vi "RespaceForSP.vi"(9 "Keep spaces?":bool, 11 "Code":string) -> (3 "Cleaned for SPIKE":string)   [LabVIEW 2020]
panel:
  out "spreadsheet string":string
  out "Array":i32[](array[numeric])
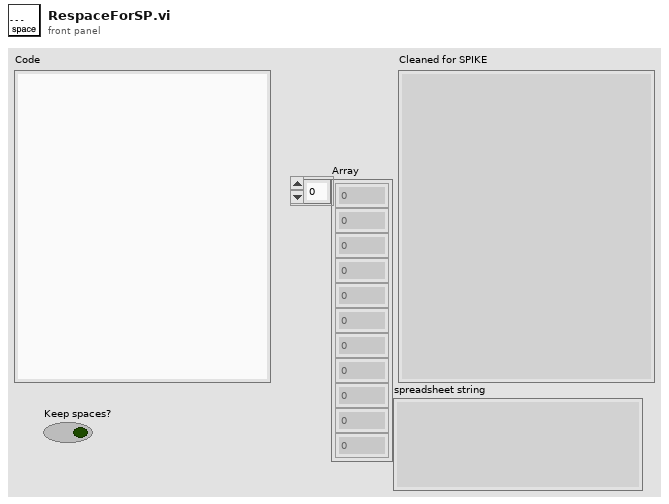
[diagram p1: front panel]
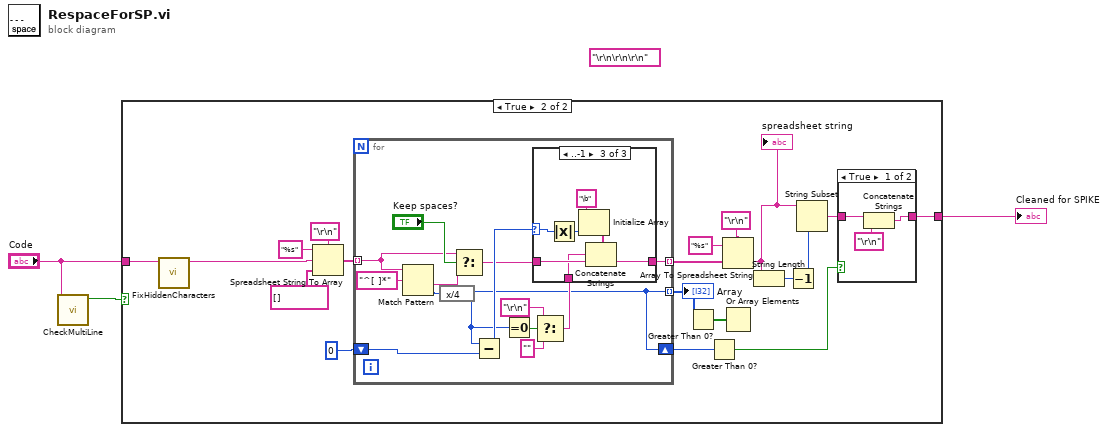
[diagram p0: block diagram]
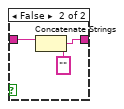
[diagram p3: hidden frame]
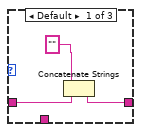
[diagram p4: hidden frame]
diagram:
  (unwired) "\r\n\r\n\r\n" ("replace string (\"\")")
  n1 = call "CheckMultiLine.vi"("Code"="Code") -> ("MultiLine?"=w1:bool)  [unwired: 10 in]
  n2 = case shown="True" w1 {
    tunnel: "Code" -> [w4 w23]
    tunnel: [w4 w14] -> w3
    frame False {
    }
    frame True {
      n3 = call "FixHiddenCharacters.vi"("String in"=w23) -> ("String out"=w5:string)  [unwired: 10 in]
      n4 = Spreadsheet String To Array(delimiter (Tab)="\r\n" ("replace string (\"\")"), format string="%s", spreadsheet string=w5, array type (2D Dbl)=string[] []) -> (array=w19:string[])
      n5 = for {
        tunnel: [w31] -> _ mode=indexing
        tunnel: w19 -> [w31] mode=indexing
        tunnel: [w34] -> w13 mode=indexing
        tunnel: [w40] -> w18 mode=indexing
        shift-right: [w34] -> w7
        shift-left: 0 ("offset past match") -> [w42]
        n6 = Match Pattern(string=w31, regular expression="^[ ]*") -> (after substring=w32:string, offset past match=w35:i32)  [unwired: 1 in, 2 out]
        n7 = expression code="x/4"(w35) -> (w34:i32)
        n8 = Select(t=w31, s="Keep spaces?", f=w32) -> (s? t:f=w30:string)
        n9 = Subtract(x=w34, y=w42) -> (x-y=w41:i32)
        n10 = Equal To 0?(x=w34) -> (x = 0?=w39:bool)
        n11 = Select(t="\r\n" ("replace string (\"\")"), s=w39, f="" ("replace string (\"\")")) -> (s? t:f=w36:string)
        n12 = case shown="..-1" w41 {
          selector: w41 -> [_ _ w52]
          tunnel: [w45 w47 w54] -> w40
          tunnel: w30 -> [w46 w47 w53]
          tunnel: w36 -> [_ _ w48]
          frame Default {
            n13 = Concatenate Strings("" ("replace string (\"\")"), w46) -> (w45:string)
          }
          frame 0 {
          }
          frame ..-1 {
            n14 = Absolute Value(x=w52) -> (abs(x)=w50:i32)
            n15 = Initialize Array("\b" ("replace string (\"\")"), w50) -> (w49:string[])
            n16 = Concatenate Strings(w49, w48, w53) -> (w54:string)
          }
        }
      }
      "Array" <- w13
      n17 = Greater Than 0?(x=w13) -> (x > 0?=w12:bool[])
      n18 = Greater Than 0?(x=w7) -> (x > 0?=w6:bool)
      n19 = Array To Spreadsheet String(delimiter (Tab)="\r\n" ("replace string (\"\")"), array=w18, 3:"%s" ("format string")) -> (spreadsheet string=w10:string)
      "spreadsheet string" <- w10
      n20 = Or Array Elements(Boolean array=w12) -> ()  [unwired: 1 out]
      n21 = String Length(string=w10) -> (length=w11:i32)
      n22 = Decrement(x=w11) -> (x-1=w8:i32)
      n23 = String Subset(string=w10, length (rest)=w8) -> (substring=w9:string)  [unwired: 1 in]
      n24 = case shown="True" w6 {
        tunnel: w9 -> [w25 w28]
        tunnel: [w24 w27] -> w14
        frame True {
          n25 = Concatenate Strings(w25, "\r\n" ("replace string (\"\")")) -> (w24:string)
        }
        frame False {
          n26 = Concatenate Strings(w28, "" ("replace string (\"\")")) -> (w27:string)
        }
      }
    }
  }
  "Cleaned for SPIKE" <- w3
